vi "getBSONValueFromName.vi"(8 "error in (no error)":errorcluster, 9 "Cluster Type (optional)":variant, 10 "Element Name":string, 11 "tBSONDocument in":refnum<class "tBSONDocument.lvclass">) -> (0 "error out":errorcluster, 2 "Variant":variant, 3 "tBSONDocument out":refnum<class "tBSONDocument.lvclass">)   [LabVIEW 2013, in "BSON.lvlib" / "tBSONDocument.lvclass"]
uses:
  tBSONDocument.lvclass
  tBSONElement/tBSONElement.lvclass
  getBooleanValue.vi
  getDoubleValue.vi
  getI32Value.vi
  getI64Value.vi
  getDocumentValue.vi
  getTimestampValue.vi
  getStringValue.vi
  getObjectIDValue.vi
  getBinaryValue.vi
  getRegExValue.vi
  getJavaScriptValue.vi
  getArrayValue.vi
  addDocumentElement.vi
  <vilib>/Utility/VariantDataType/VariantType.lvlib
  BSON.lvlib
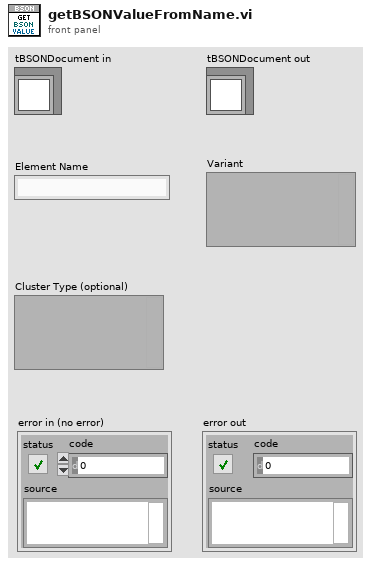
[diagram p1: front panel]
types:
  T1 = typedef "VariantType.lvlib/Type.ctl" = enum8{"Invalid Type", "Void", "I8", "I16", "I32", "I64", "U8", "U16", "U32", "U64", "Single Float", "Double Float", "Extended Float", "Single Complex", "Double Complex", "Extended Complex", "Enum U8", "Enum U16", "Enum U32", "Enum U64", "Single Float With Unit", "Double Float With Unit", "Extended Float With Unit", "Single Complex with Unit", "Double Complex with Unit", "Extended Complex with Unit", "Boolean", "String", "Path", "Picture", "Tag", "Array", "Cluster", "Variant", "LV Variant", "Waveform", "Timestamp", "Digital Waveform", "Digital Data", "ExpressData", "Refnum", "External Data", "VI", "Poly VI", "LabVIEW Class Instance", "Fixed Point"}
  T2 = typedef "BSON.lvlib/tBSONElement.lvclass/type.ctl" = u8
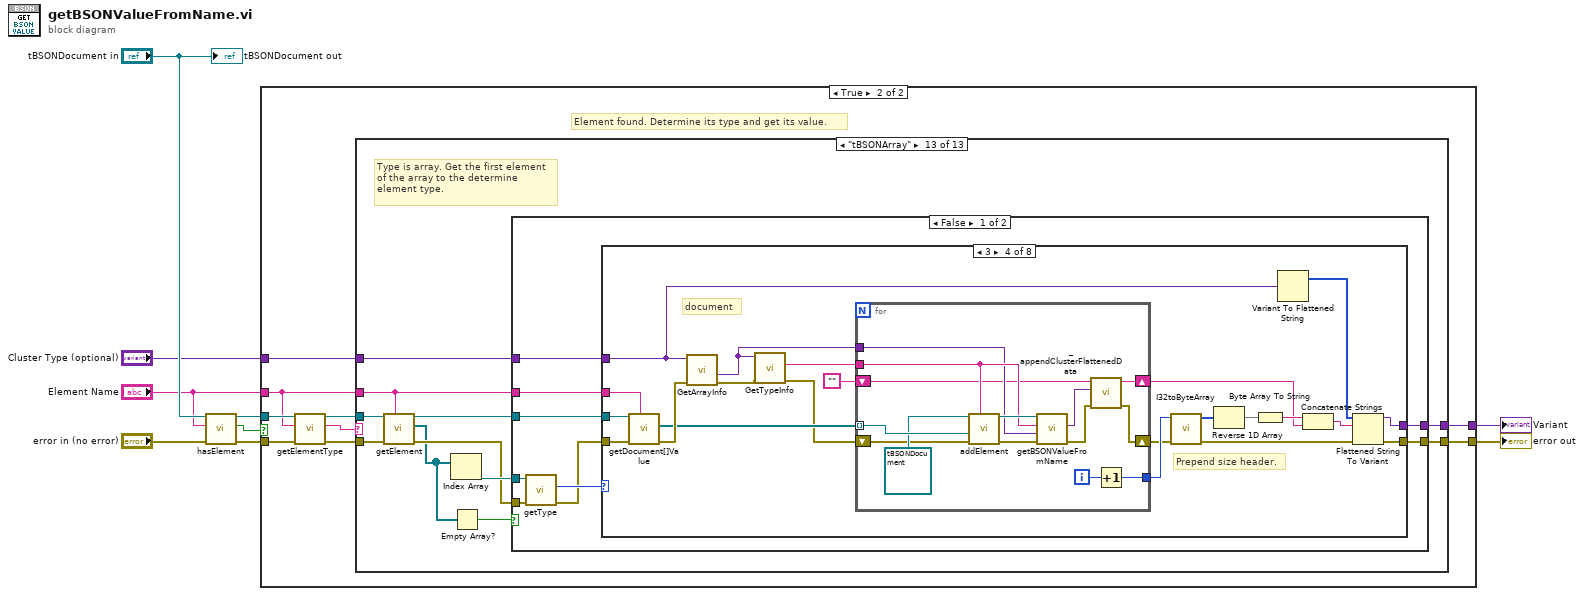
[diagram p0: block diagram]
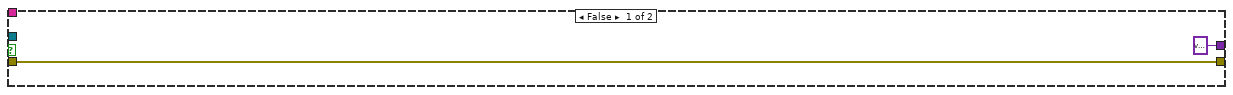
[diagram p2: hidden frame]
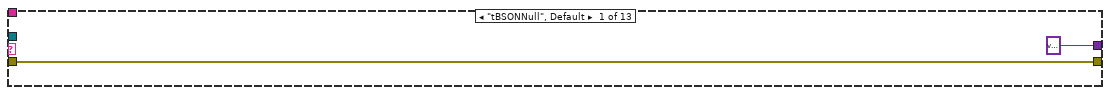
[diagram p3: hidden frame]
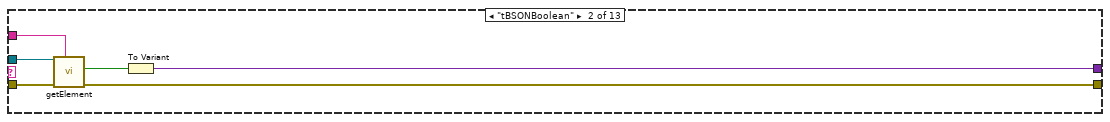
[diagram p4: hidden frame]
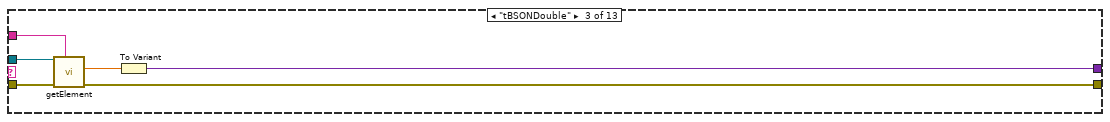
[diagram p5: hidden frame]
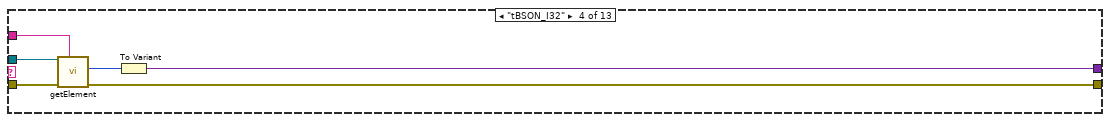
[diagram p6: hidden frame]
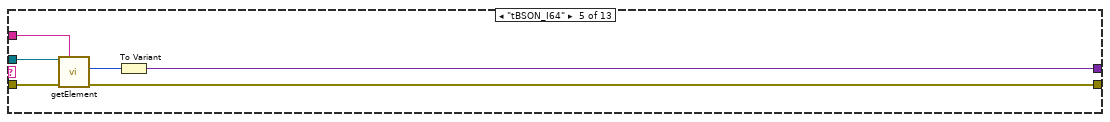
[diagram p7: hidden frame]
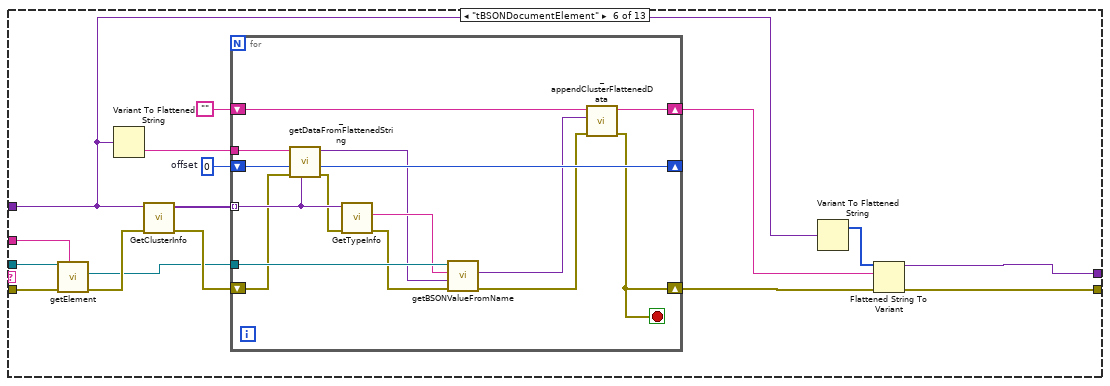
[diagram p8: hidden frame]
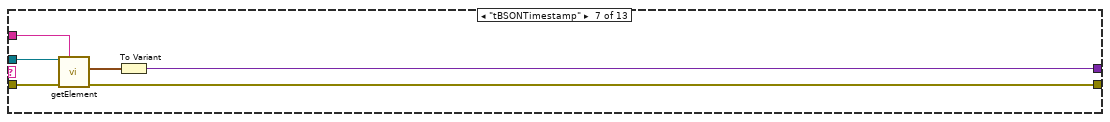
[diagram p9: hidden frame]
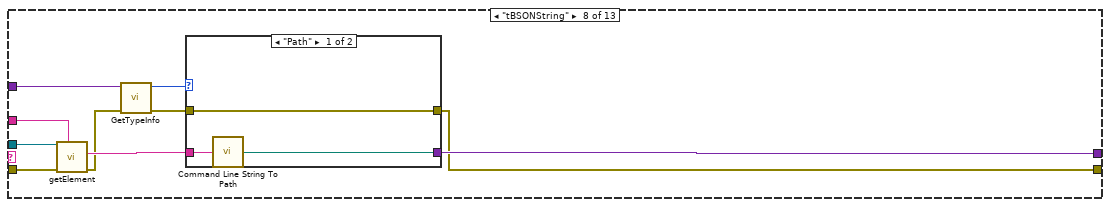
[diagram p10: hidden frame]
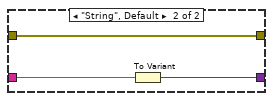
[diagram p11: hidden frame]
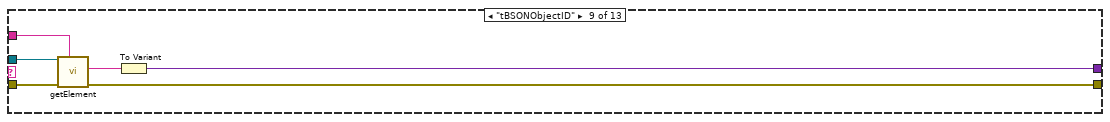
[diagram p12: hidden frame]
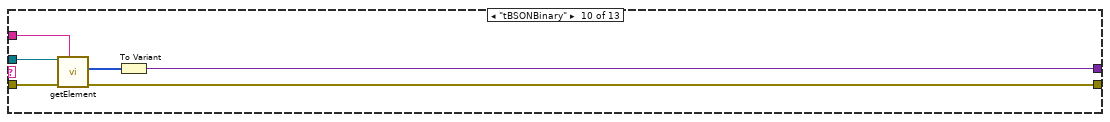
[diagram p13: hidden frame]
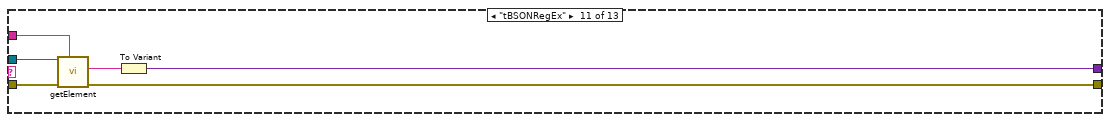
[diagram p14: hidden frame]
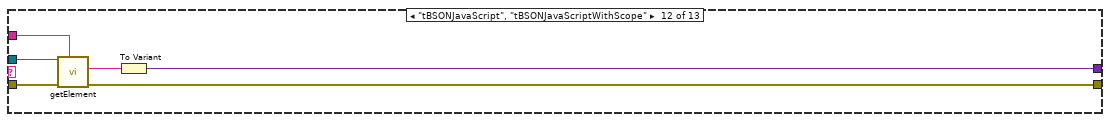
[diagram p15: hidden frame]
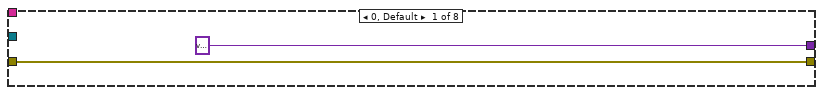
[diagram p16: hidden frame]
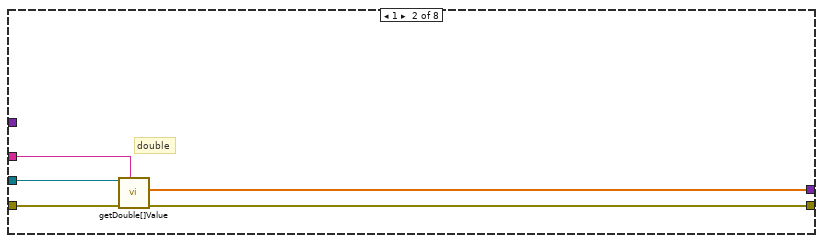
[diagram p17: hidden frame]
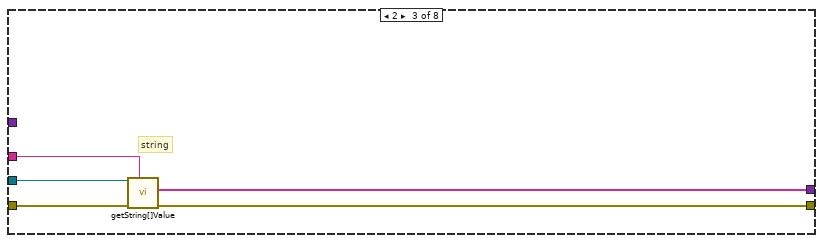
[diagram p18: hidden frame]
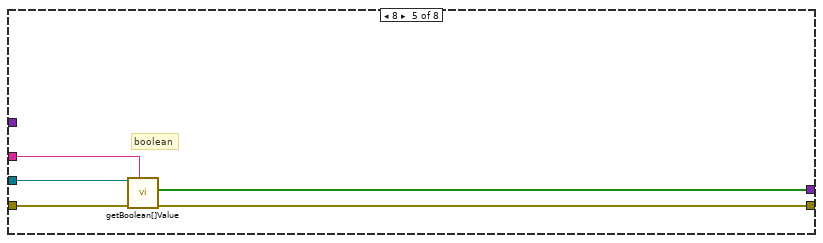
[diagram p19: hidden frame]
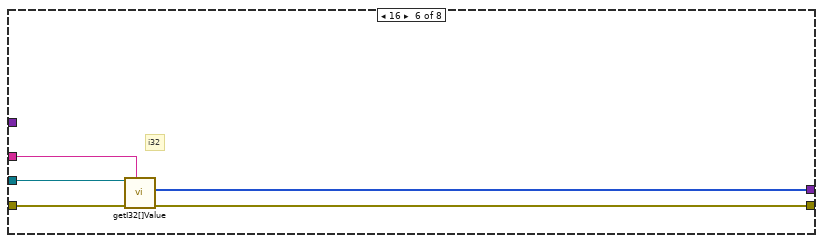
[diagram p20: hidden frame]
diagram:
  n1 = call "hasElement.vi"("error in (no error)"="error in (no error)", "Name"="Element Name", "tBSONDocument in"="tBSONDocument in") -> ("error out"=w3:errorcluster, "hasElement"=w4:bool, "tBSONDocument out"=w6:refnum<class "tBSONDocument.lvclass">)  [unwired: 6 in]
  n2 = case shown="True" w4 {
    tunnel: w6 -> [_ w18]
    tunnel: w3 -> [w11 w16]
    tunnel: [w11 w20] -> w9
    tunnel: "Element Name" -> [_ w13]
    tunnel: [variant ("Variant") w19] -> w8
    tunnel: "Cluster Type (optional)" -> [_ w12]
    frame False {
    }
    frame True {
      # "Element found. Determine its type and get its value."
      n3 = call "getElementType.vi"("error in (no error)"=w16, "Name"=w13, "tBSONDocument in"=w18) -> ("error out"=w15:errorcluster, "TypeClass"=w14:string, "tBSONDocument out"=w17:refnum<class "tBSONDocument.lvclass">)  [unwired: 6 in]
      n4 = case shown="\"tBSONArray\"" w14 {
        tunnel: w17 -> [_ w27 w33 w38 w45 w61 w82 w91 w103 w110 w115 w122 w132]
        tunnel: w15 -> [w22 w23 w31 w37 w43 w60 w81 w90 w102 w108 w114 w118 w131]
        tunnel: w13 -> [_ w26 w32 w39 w44 w62 w80 w92 w104 w109 w116 w121 w129]
        tunnel: [w22 w24 w29 w36 w42 w48 w78 w84 w101 w107 w113 w119 w133] -> w20
        tunnel: [variant ("Variant") w28 w34 w40 w46 w47 w83 w93 w105 w111 w117 w123 w134] -> w19
        tunnel: w12 -> [_ _ _ _ _ w51 _ w88 _ _ _ _ w128]
        frame "tBSONNull", Default {
        }
        frame "tBSONBoolean" {
          n5 = call-poly "getElement.vi"("Name"=w26, "error in (no error)"=w23, "tBSONDocument in"=w27) -> ("error out"=w24:errorcluster, "Value"=w25:bool)  [unwired: 6 in, 1 out]
          n6 = To Variant(anything=w25) -> (Variant=w28:variant)
        }
        frame "tBSONDouble" {
          n7 = call-poly "getElement.vi"("Name"=w32, "error in (no error)"=w31, "tBSONDocument in"=w33) -> ("error out"=w29:errorcluster, "Value"=w30:dbl)  [unwired: 6 in, 1 out]
          n8 = To Variant(anything=w30) -> (Variant=w34:variant)
        }
        frame "tBSON_I32" {
          n9 = call-poly "getElement.vi"("Name"=w39, "error in (no error)"=w37, "tBSONDocument in"=w38) -> ("error out"=w36:errorcluster, "Value"=w35:i32)  [unwired: 6 in, 1 out]
          n10 = To Variant(anything=w35) -> (Variant=w40:variant)
        }
        frame "tBSON_I64" {
          n11 = call-poly "getElement.vi"("Name"=w44, "error in (no error)"=w43, "tBSONDocument in"=w45) -> ("error out"=w42:errorcluster, "Value"=w41:i64)  [unwired: 6 in, 1 out]
          n12 = To Variant(anything=w41) -> (Variant=w46:variant)
        }
        frame "tBSONDocumentElement" {
          w55 = 0  # offset
          n13 = call-poly "getElement.vi"("Name"=w62, "error in (no error)"=w60, "tBSONDocument in"=w61) -> ("error out"=w59:errorcluster, "Value"=w56:refnum<class "tBSONDocument.lvclass">)  [unwired: 6 in, 1 out]
          n14 = Variant To Flattened String(Variant=w51) -> (data string=w54:string)  [unwired: 1 out]
          n15 = call <vilib>:"GetClusterInfo.vi"("error in (no error)"=w59, "Variant"=w51) -> ("error out"=w58:errorcluster, "Cluster Elements"=w57:variant[])  [unwired: 8 in]
          n16 = for {
            tunnel: w57 -> [w72] mode=indexing
            tunnel: w56 -> [w77]
            shift-right: [w64] -> w49
            shift-left: w58 -> [w71]
            shift-right: [w69] -> _
            shift-left: w55 -> [w73]
            tunnel: w54 -> [w74]
            shift-right: [w63] -> w52
            shift-left: "" -> [w67]
            stop <- w64 stop-if-true
            n17 = call "_getDataFromFlattenedString.vi"("type descriptor"=w72, "error in (no error)"=w71, "offset to extract data"=w73, "flattened data"=w74) -> ("error out"=w70:errorcluster, "offset past data"=w69:i32, "data"=w68:variant)  [unwired: 5 in]
            n18 = call <vilib>:"GetTypeInfo.vi"("error in (no error)"=w70, "Variant"=w72) -> ("error out"=w75:errorcluster, "Name"=w76:string)  [unwired: 5 in, 3 out]
            n19 = call "getBSONValueFromName.vi"("error in (no error)"=w75, "Cluster Type (optional)"=w68, "Element Name"=w76, "tBSONDocument in"=w77) -> ("error out"=w65:errorcluster, "Variant"=w66:variant)  [unwired: 5 in, 1 out]
            n20 = call "_appendClusterFlattenedData.vi"("error in (no error)"=w65, "Variant Data"=w66, "Flattened Cluster"=w67) -> ("error out"=w64:errorcluster, "Appended Cluster"=w63:string)  [unwired: 7 in]
          }
          n21 = Variant To Flattened String(Variant=w51) -> (1:w50:i16[])  [unwired: 1 out]
          n22 = Flattened String To Variant(4:w49, 6:w52, 7:w50) -> (0:w48:errorcluster, 3:w47:variant)
        }
        frame "tBSONTimestamp" {
          n23 = call-poly "getElement.vi"("Name"=w80, "error in (no error)"=w81, "tBSONDocument in"=w82) -> ("error out"=w78:errorcluster, "Value"=w79:timestamp)  [unwired: 6 in, 1 out]
          n24 = To Variant(anything=w79) -> (Variant=w83:variant)
        }
        frame "tBSONString" {
          n25 = call-poly "getElement.vi"("Name"=w92, "error in (no error)"=w90, "tBSONDocument in"=w91) -> ("error out"=w87:errorcluster, "Value"=w89:string)  [unwired: 6 in, 1 out]
          n26 = call <vilib>:"GetTypeInfo.vi"("error in (no error)"=w87, "Variant"=w88) -> ("error out"=w86:errorcluster, "Type Enum"=w85:T1)  [unwired: 5 in, 3 out]
          n27 = case shown="\"Path\"" w85 {
            tunnel: [w95 w99] -> w93
            tunnel: w89 -> [w96 w98]
            tunnel: w86 -> [w94 w97]
            tunnel: [w94 w97] -> w84
            frame "Path" {
              n28 = call <vilib>:"Command Line String To Path.vi"("string"=w96) -> ("path"=w95:path)
            }
            frame "String", Default {
              n29 = To Variant(anything=w98) -> (Variant=w99:variant)
            }
          }
        }
        frame "tBSONObjectID" {
          n30 = call-poly "getElement.vi"("Name"=w104, "error in (no error)"=w102, "tBSONDocument in"=w103) -> ("error out"=w101:errorcluster, "Value"=w100:string)  [unwired: 6 in, 1 out]
          n31 = To Variant(anything=w100) -> (Variant=w105:variant)
        }
        frame "tBSONBinary" {
          n32 = call-poly "getElement.vi"("Name"=w109, "error in (no error)"=w108, "tBSONDocument in"=w110) -> ("error out"=w107:errorcluster, "Value"=w106:u8[])  [unwired: 6 in, 1 out]
          n33 = To Variant(anything=w106) -> (Variant=w111:variant)
        }
        frame "tBSONRegEx" {
          n34 = call-poly "getElement.vi"("Name"=w116, "error in (no error)"=w114, "tBSONDocument in"=w115) -> ("error out"=w113:errorcluster, "RegEx"=w112:string)  [unwired: 5 in, 2 out]
          n35 = To Variant(anything=w112) -> (Variant=w117:variant)
        }
        frame "tBSONJavaScript", "tBSONJavaScriptWithScope" {
          n36 = call-poly "getElement.vi"("Name"=w121, "error in (no error)"=w118, "tBSONDocument in"=w122) -> ("error out"=w119:errorcluster, "Value"=w120:string)  [unwired: 6 in, 1 out]
          n37 = To Variant(anything=w120) -> (Variant=w123:variant)
        }
        frame "tBSONArray" {
          # "Type is array. Get the first element\nof the array to the determine\nelement type."
          n38 = call-poly "getElement.vi"("Name"=w129, "error in (no error)"=w131, "tBSONDocument in"=w132) -> ("error out"=w126:errorcluster, "Value"=w125:refnum<class "tBSONElement.lvclass">[], "tBSONDocument out"=w130:refnum<class "tBSONDocument.lvclass">)  [unwired: 6 in]
          n39 = Index Array(array=w125) -> (element=w127:refnum<class "tBSONElement.lvclass">)  [unwired: 1 in]
          n40 = Empty Array?(array=w125) -> (empty?=w124:bool)
          n41 = case shown="False" w124 {
            tunnel: [w141 w218] -> w134
            tunnel: [w140 w219] -> w133
            tunnel: w130 -> [w139 _]
            tunnel: w129 -> [w138 _]
            tunnel: w128 -> [w137 w212]
            tunnel: w127 -> [w136 _]
            tunnel: w126 -> [w135 w216]
            frame False {
              n42 = call-dynamic "getType.vi"("error in (no error)"=w135, "tBSONElement in"=w136) -> ("error out"=w142:errorcluster, "Type"=w143:T2)  [unwired: 7 in, 1 out]
              n43 = case shown="3" w143 {
                tunnel: w142 -> [w144 w149 w152 w176 w195 w199 w205 w210]
                tunnel: w139 -> [_ w150 w155 w177 w196 w201 w206 w211]
                tunnel: [variant ("Variant") w146 w154 w156 w192 w197 w204 w208] -> w141
                tunnel: [w144 w148 w153 w162 w193 w198 w203 w209] -> w140
                tunnel: w138 -> [_ w147 w151 w175 w194 w200 w202 w207]
                tunnel: w137 -> [_ _ _ w163 _ _ _ _]
                frame 0, Default {
                }
                frame 1 {
                  # "double"
                  n44 = call "getDouble[]Value.vi"("Name"=w147, "error in (no error)"=w149, "tBSONDocument in"=w150) -> ("error out"=w148:errorcluster, "Value"=w146:dbl[])  [unwired: 6 in, 1 out]
                }
                frame 2 {
                  # "string"
                  n45 = call "getString[]Value.vi"("Name"=w151, "error in (no error)"=w152, "tBSONDocument in"=w155) -> ("error out"=w153:errorcluster, "Value"=w154:string[])  [unwired: 6 in, 1 out]
                }
                frame 3 {
                  # "Prepend size header."
                  # "document"
                  n46 = call "getDocument[]Value.vi"("Name"=w175, "error in (no error)"=w176, "tBSONDocument in"=w177) -> ("error out"=w174:errorcluster, "Value"=w173:refnum<class "tBSONDocument.lvclass">[])  [unwired: 6 in, 1 out]
                  n47 = call <vilib>:"GetArrayInfo.vi"("error in (no error)"=w174, "Variant"=w163) -> ("error out"=w171:errorcluster, "ArrayElement"=w169:variant)  [unwired: 6 in, 2 out]
                  n48 = call <vilib>:"GetTypeInfo.vi"("error in (no error)"=w171, "Variant"=w169) -> ("error out"=w170:errorcluster, "Name"=w172:string)  [unwired: 5 in, 3 out]
                  n49 = for {
                    shift-right: [w178] -> w166
                    shift-left: w170 -> [w186]
                    tunnel: w173 -> [w191] mode=indexing
                    tunnel: w172 -> [w187]
                    tunnel: w169 -> [w185]
                    shift-right: [w182] -> w160
                    shift-left: "" -> [w181]
                    tunnel: [w183] -> w167
                    i -> [w184]
                    n50 = call-poly "addElement.vi"("Name"=w187, "error in (no error)"=w186, "Value"=w191, "tBSONDocument in"=refnum<class "tBSONDocument.lvclass"> refnum) -> ("error out"=w188:errorcluster, "tBSONDocument out"=w189:refnum<class "tBSONDocument.lvclass">)  [unwired: 6 in]
                    n51 = call "getBSONValueFromName.vi"("error in (no error)"=w188, "Cluster Type (optional)"=w185, "Element Name"=w187, "tBSONDocument in"=w189) -> ("error out"=w179:errorcluster, "Variant"=w180:variant)  [unwired: 5 in, 1 out]
                    n52 = call "_appendClusterFlattenedData.vi"("error in (no error)"=w179, "Variant Data"=w180, "Flattened Cluster"=w181) -> ("error out"=w178:errorcluster, "Appended Cluster"=w182:string)  [unwired: 7 in]
                    n53 = Increment(x=w184) -> (x+1=w183:i32)
                  }
                  n54 = call "I32toByteArray.vi"("error in (no error)"=w166, "I32"=w167) -> ("error out"=w157:errorcluster, "LittleEndianByteArray"=w165:u8[])  [unwired: 8 in]
                  n55 = Reverse 1D Array(array=w165) -> (reversed array=w164:u8[])
                  n56 = Byte Array To String(unsigned byte array=w164) -> (string=w161:string)
                  n57 = Variant To Flattened String(Variant=w163) -> (1:w158:i16[])  [unwired: 1 out]
                  n58 = Concatenate Strings(w161, w160) -> (w159:string)
                  n59 = Flattened String To Variant(4:w157, 6:w159, 7:w158) -> (0:w162:errorcluster, 3:w156:variant)
                }
                frame 8 {
                  # "boolean"
                  n60 = call "getBoolean[]Value.vi"("Name"=w194, "error in (no error)"=w195, "tBSONDocument in"=w196) -> ("error out"=w193:errorcluster, "Value"=w192:bool[])  [unwired: 6 in, 1 out]
                }
                frame 16 {
                  # "i32"
                  n61 = call "getI32[]Value.vi"("Name"=w200, "error in (no error)"=w199, "tBSONDocument in"=w201) -> ("error out"=w198:errorcluster, "Value"=w197:i32[])  [unwired: 6 in, 1 out]
                }
                frame 17 {
                  # "timestamp"
                  n62 = call "getTimestamp[]Value.vi"("Name"=w202, "error in (no error)"=w205, "tBSONDocument in"=w206) -> ("error out"=w203:errorcluster, "Value"=w204:timestamp[])  [unwired: 6 in, 1 out]
                }
                frame 18 {
                  # "i64"
                  n63 = call "getI64[]Value.vi"("Name"=w207, "error in (no error)"=w210, "tBSONDocument in"=w211) -> ("error out"=w209:errorcluster, "Value"=w208:i64[])  [unwired: 6 in, 1 out]
                }
              }
            }
            frame True {
              n64 = call <vilib>:"GetArrayInfo.vi"("error in (no error)"=w216, "Variant"=w212) -> ("error out"=w215:errorcluster, "ArrayElement"=w214:variant)  [unwired: 6 in, 2 out]
              n65 = Initialize Array(w214, 0 ("dimension size")) -> (w213:variant[])
              n66 = Variant To Data(error in=w215, type=w212, Variant=w213) -> (data=w218:variant, error out=w219:errorcluster)
            }
          }
        }
      }
    }
  }
  "error out" <- w9
  "Variant" <- w8
  "tBSONDocument out" <- "tBSONDocument in"
